vi "waveAquis.vi"(4 "Timeout (10000 ms)":u32=10000, 5 "Sub Channel(0: None)":u16(ring) items=["None", "SCH1", "SCH2", "SCH3", "SCH4", "SCH5", "SCH6", "SCH7", "SCH8", "SCH9", "SCH10", "SCH11", "SCH12", "SCH13", "SCH14", "SCH15", "SCH16", "SCH17", "SCH18", "SCH19", "SCH20", "SCH21", "SCH22", "SCH23", "SCH24", "SCH25", "SCH26", "SCH27", "SCH28", "SCH29", "SCH30", "SCH31", "SCH32", "SCH33", "SCH34", "SCH35", "SCH36", "SCH37", "SCH38", "SCH39", "SCH40", "SCH41", "SCH42", "SCH43", "SCH44", "SCH45", "SCH46", "SCH47", "SCH48", "SCH49", "SCH50", "SCH51", "SCH52", "SCH53", "SCH54", "SCH55", "SCH56", "SCH57", "SCH58", "SCH59", "SCH60", "SCH61", "SCH62", "SCH63", "SCH64"], 6 "End Point(1000)":i64=1000, 7 "Source (1: CH1)":i32(ring)=1 items=["", "CH1", "CH2", "CH3", "CH4", "CH5", "CH6", "CH7", "CH8", "CH9", "CH10", "CH11", "CH12", "CH13", "CH14", "CH15", "CH16", "MATH1", "MATH2", "MATH3", "MATH4", "MATH5", "MATH6", "MATH7", "MATH8", "EVENT"], 8 "error in (no error)":errorcluster, 9 "Start Point(0)":i64, 10 "Record Number (0)":i32, 11 "VISA resource name":refnum<visa-resource-name>) -> (0 "error out":errorcluster, 2 "Waveform Data":waveform(dbl)(graph), 3 "VISA resource name out":refnum<visa-resource-name>)   [LabVIEW 2019]
panel:
  out "read buffer":string
  out "output 2":dbl
  out "output 1":dbl
  out "1/x":dbl
  out "error out 9":errorcluster
  out "error out 8":errorcluster
  out "error out 7":errorcluster
  out "error out 6":errorcluster
  out "error out 5":errorcluster
  out "error out 4":errorcluster
  out "error out 3":errorcluster
  out "result":bool
  out "error out 2":errorcluster
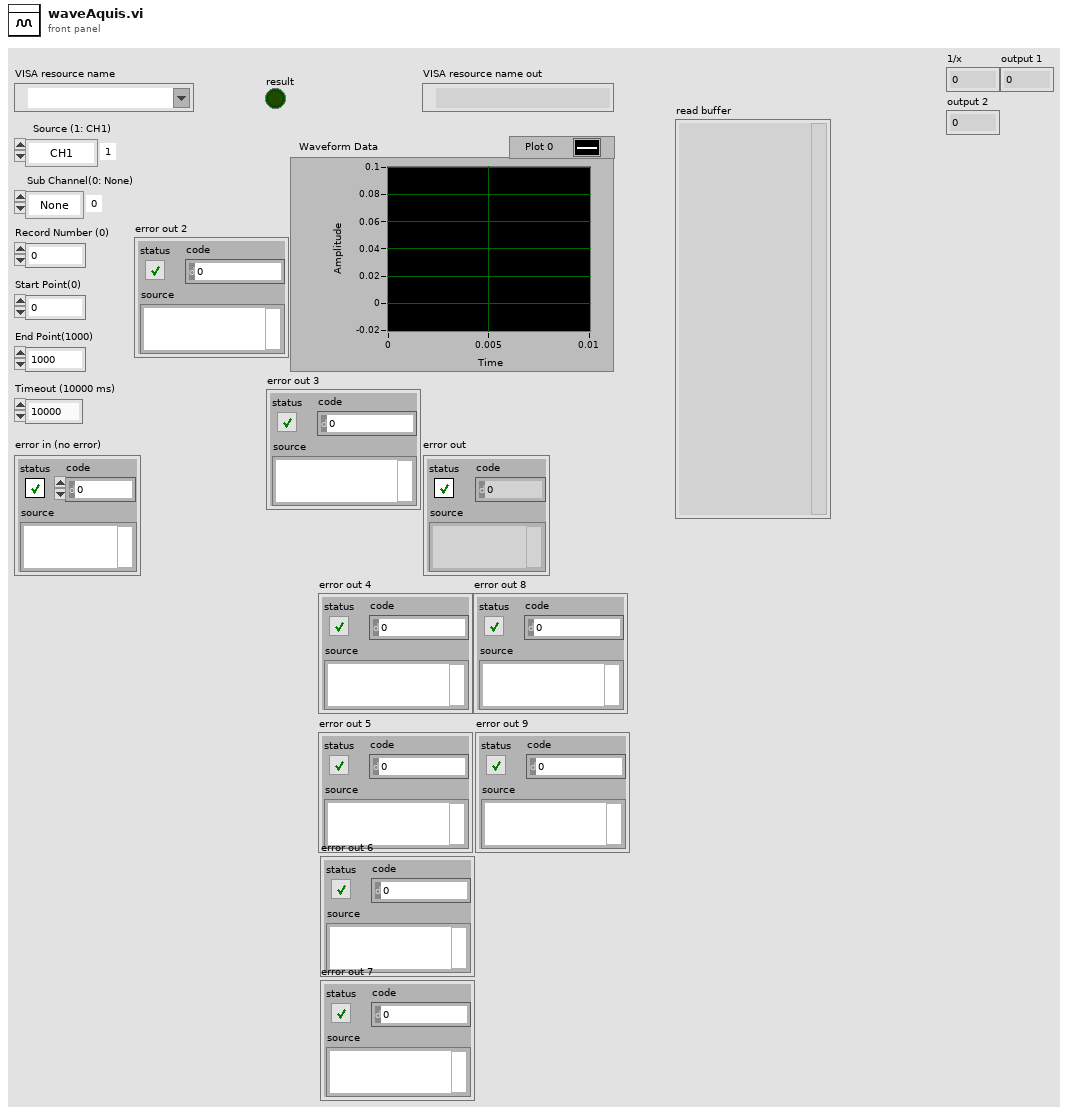
[diagram p1: front panel]
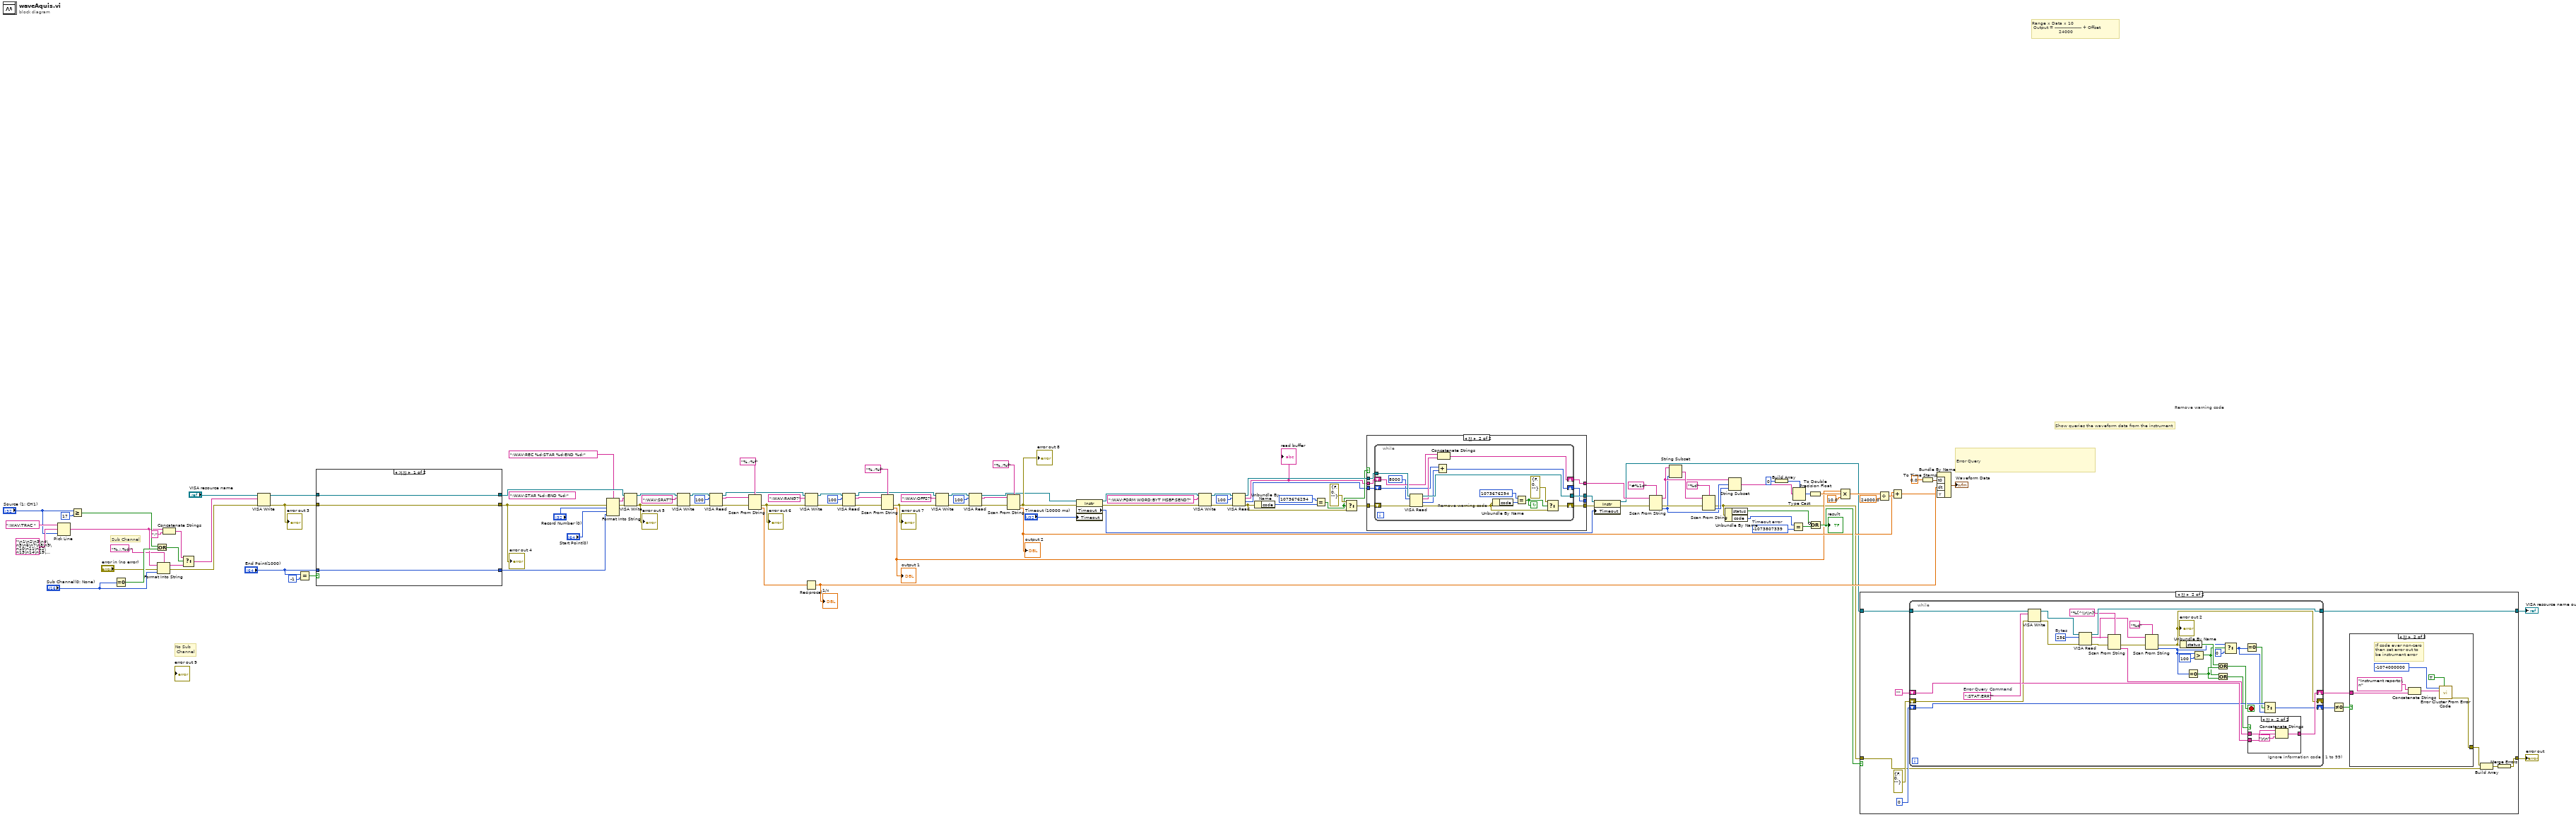
[diagram p0: block diagram]
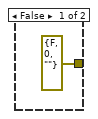
[diagram p4: hidden frame]
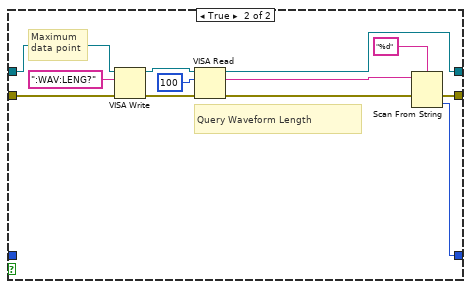
[diagram p6: hidden frame]
diagram:
  w61 = -1073807339  # Timeout error
  (unwired) ":WAV:STAR %d;:END %d;"
  # "Remove warning code"
  # "Show queries the waveform data from the instrument"
  # "Range x Data x 10\n Output = ------------------- + Offset \n                   24000"
  # "Error Query"
  # "Sub Channel"
  # "No Sub\n Channel"
  n1 = Pick Line ("ライン選択")(string ("")=":WAV:TRAC ", multi-line string="\n1\n2\n3\n4\n5\n6\n7\n8\n9\n10\n11\n12\n13\n14\n15\n16\nMATH1\nMATH2\nMATH3\nMATH4\nMATH5\nMATH6\nMATH7\nMATH8\nEVEN", line index="Source (1: CH1)") -> (output string=w95:string)
  n2 = Greater Or Equal? ("Èã?")(x="Source (1: CH1)", y=u16 17) -> (x >= y?=w109:bool)
  n3 = Equal To 0? ("0に等しい?")(x="Sub Channel(0: None)") -> (x = 0?=w110:bool)
  n4 = Or(x=w109, y=w110) -> (x .or. y?=w96:bool)
  n5 = Format Into String ("文字列にフォーマット")(format string="%.;,%d;", initial string=w95, error in="error in (no error)", "Sub Channel(0: None)") -> (resulting string=w93:string, error out=w101:errorcluster)
  n6 = Concatenate Strings ("•¶Žš—ñ˜AŒ‹")(w95, ";") -> (w97:string)
  n7 = Select(t=w97, s=w96, f=w93) -> (s? t:f=w92:string)
  n8 = VISA Write ("VISA書き込み")(VISA resource name="VISA resource name", write buffer=w92, error in (no error)=w101) -> (VISA resource name out=w100:refnum<visa-resource-name>, error out=w99:errorcluster)  [unwired: 1 out]
  "error out 3" <- w99
  n9 = Equal?(x="End Point(1000)", y=-1) -> (x = y?=w105:bool)
  n10 = case shown="거짓" w105 {
    tunnel: w100 -> [w115 w121]
    tunnel: [w115 w119] -> w104
    tunnel: [w116 w117] -> w103
    tunnel: "End Point(1000)" -> [w116 _]
    tunnel: w99 -> [w114 w120]
    tunnel: [w114 w118] -> w55
    frame False {
    }
    frame True {
      # "Query Waveform Length"
      # "Maximum\ndata point"
      n11 = VISA Write ("VISA書き込み")(VISA resource name=w121, write buffer=":WAV:LENG?", error in (no error)=w120) -> (VISA resource name out=w127:refnum<visa-resource-name>, error out=w128:errorcluster)  [unwired: 1 out]
      n12 = VISA Read ("VISA読み取り")(VISA resource name=w127, byte count=u32 100, error in (no error)=w128) -> (VISA resource name out=w119:refnum<visa-resource-name>, read buffer=w123:string, error out=w122:errorcluster)  [unwired: 1 out]
      n13 = Scan From String ("文字列からスキャン")(format string="%d", input string=w123, error in=w122) -> (error out=w118:errorcluster, output 1=w117:i32)  [unwired: 2 in, 2 out]
    }
  }
  "error out 4" <- w55
  n14 = Format Into String ("文字列にフォーマット")(format string=":WAV:REC %d;STAR %d;END %d;", error in=w55, "Record Number (0)", "Start Point(0)", w103) -> (resulting string=w4:string, error out=w5:errorcluster)  [unwired: 1 in]
  n15 = VISA Write ("VISA書き込み")(VISA resource name=w104, write buffer=w4, error in (no error)=w5) -> (VISA resource name out=w63:refnum<visa-resource-name>, error out=w54:errorcluster)  [unwired: 1 out]
  "error out 5" <- w54
  n16 = VISA Write ("VISA書き込み")(VISA resource name=w63, write buffer=":WAV:SRAT?", error in (no error)=w54) -> (VISA resource name out=w84:refnum<visa-resource-name>, error out=w86:errorcluster)  [unwired: 1 out]
  n17 = VISA Read ("VISA読み取り")(VISA resource name=w84, byte count=u32 100, error in (no error)=w86) -> (VISA resource name out=w62:refnum<visa-resource-name>, read buffer=w80:string, error out=w79:errorcluster)  [unwired: 1 out]
  n18 = Scan From String ("文字列からスキャン")(format string="%.;%f", input string=w80, error in=w79) -> (error out=w53:errorcluster, output 1=w81:dbl)  [unwired: 2 in, 2 out]
  "error out 6" <- w53
  n19 = VISA Write ("VISA書き込み")(VISA resource name=w62, write buffer=":WAV:RANG?", error in (no error)=w53) -> (VISA resource name out=w76:refnum<visa-resource-name>, error out=w77:errorcluster)  [unwired: 1 out]
  n20 = Reciprocal ("t")(x=w81) -> (1/x=w78:dbl)
  "1/x" <- w78
  n21 = VISA Read ("VISA読み取り")(VISA resource name=w76, byte count=u32 100, error in (no error)=w77) -> (VISA resource name out=w56:refnum<visa-resource-name>, read buffer=w72:string, error out=w71:errorcluster)  [unwired: 1 out]
  n22 = Scan From String(format string="%.;%f", input string=w72, error in=w71) -> (error out=w52:errorcluster, output 1=w34:dbl)  [unwired: 2 in, 2 out]
  "error out 7" <- w52
  "output 1" <- w34
  n23 = VISA Write ("VISA書き込み")(VISA resource name=w56, write buffer=":WAV:OFFS?", error in (no error)=w52) -> (VISA resource name out=w68:refnum<visa-resource-name>, error out=w70:errorcluster)  [unwired: 1 out]
  n24 = VISA Read ("VISA読み取り")(VISA resource name=w68, byte count=u32 100, error in (no error)=w70) -> (VISA resource name out=w17:refnum<visa-resource-name>, read buffer=w65:string, error out=w64:errorcluster)  [unwired: 1 out]
  n25 = Scan From String ("文字列からスキャン")(format string="%.;%f", input string=w65, error in=w64) -> (error out=w32:errorcluster, output 1=w35:dbl)  [unwired: 2 in, 2 out]
  "error out 8" <- w32
  "output 2" <- w35
  n26 = property on="プロパティノード" class="Instr"(reference=w17, error in=w32, "Timeout"="Timeout (10000 ms)") -> (reference out=w16:refnum<visa-resource-name>, error out=w11:errorcluster, "Timeout"=w33:u32)
  n27 = VISA Write(VISA resource name=w16, write buffer=":WAV:FORM WORD;BYT MSBF;SEND?", error in (no error)=w11) -> (VISA resource name out=w31:refnum<visa-resource-name>, error out=w30:errorcluster)  [unwired: 1 out]
  n28 = VISA Read(VISA resource name=w31, byte count=u32 100, error in (no error)=w30) -> (VISA resource name out=w29:refnum<visa-resource-name>, read buffer=w20:string, return count=w21:u32, error out=w24:errorcluster)
  "read buffer" <- w20
  n29 = Unbundle By Name(w24) -> ("code"=w28:i32)
  n30 = Equal?(x=1073676294, y=w28) -> (x = y?=w23:bool)
  n31 = Select(t=errorcluster {"status"=FALSE, "code"=0, "source"=""}, s=w23, f=w24) -> (s? t:f=w25:errorcluster)
  n32 = case shown="참" w23 {
    tunnel: w29 -> [w132 w140]
    tunnel: w25 -> [w131 w137]
    tunnel: [w132 w139] -> w19
    tunnel: [w131 w138] -> w18
    tunnel: w21 -> [w129 w136]
    tunnel: [w130 w135] -> w14
    tunnel: w20 -> [w130 w134]
    tunnel: [w129 w133] -> _
    frame False {
    }
    frame True {
      n33 = while {
        shift-left: w137 -> [w151]
        shift-right: [w142] -> w138
        shift-left: w134 -> [w153]
        shift-right: [w154] -> w135
        shift-left: w136 -> [w150]
        shift-right: [w148] -> w133
        tunnel: [w155] -> w139
        tunnel: w140 -> [w156]
        stop <- w141 continue-if-true
        # "Remove warning code"
        n34 = VISA Read(VISA resource name=w156, byte count=u32 8000, error in (no error)=w151) -> (VISA resource name out=w155:refnum<visa-resource-name>, read buffer=w152:string, return count=w149:u32, error out=w143:errorcluster)
        n35 = Add(x=w150, y=w149) -> (x+y=w148:u32)
        n36 = Concatenate Strings(w153, w152) -> (w154:string)
        n37 = Unbundle By Name(w143) -> ("code"=w146:i32)
        n38 = Equal?(x=1073676294, y=w146) -> (x = y?=w141:bool)
        n39 = Select(t=errorcluster {"status"=FALSE, "code"=0, "source"=""}, s=w141, f=w143) -> (s? t:f=w142:errorcluster)
      }
    }
  }
  n40 = property on="プロパティノード" class="Instr"(reference=w19, error in=w18, "Timeout"=w33) -> (reference out=w10:refnum<visa-resource-name>, error out=w9:errorcluster)
  n41 = Scan From String ("文字列からスキャン")(format string="#%1d", input string=w14, error in=w9) -> (remaining string=w40:string, error out=w45:errorcluster, output 1=w39:i32)  [unwired: 2 in, 1 out]
  n42 = String Subset ("•”•ª•¶Žš—ñ")(string=w40, length (rest)=w39) -> (substring=w42:string)  [unwired: 1 in]
  n43 = Scan From String ("文字列からスキャン")(format string="%d", input string=w42, error in=w45) -> (error out=w6:errorcluster, output 1=w41:i32)  [unwired: 2 in, 2 out]
  n44 = Unbundle By Name ("名前でバンドル解除")(w6) -> ("status"=w8:bool, "code"=w7:i32)
  n45 = String Subset ("•”•ª•¶Žš—ñ")(string=w40, offset (0)=w39, length (rest)=w41) -> (substring=w50:string)
  n46 = Build Array ("”z—ñ˜AŒ‹’Ç‰Á")(i16 0) -> (w48:i16[])
  n47 = Equal? ("等しい?")(x=w7, y=w61) -> (x = y?=w60:bool)
  n48 = Type Cast ("タイプキャスト")(type=w48, x=w50) -> (*(type *) &x=w51:i16[])
  n49 = To Double Precision Float ("倍精度浮動小数に変換")(number=w51) -> (double precision float=w38:dbl[])
  n50 = Compound Arithmetic op=OR ("¡Z")(invert w8, w60) -> (w59:bool)
  "result" <- w59
  n51 = Compound Arithmetic op=MULTIPLY(w34, w38, 10.0) -> (w36:dbl[])
  n52 = case "ケースストラクチャ" shown="참" w59 {
    tunnel: [w158 w170] -> w57
    tunnel: [w157 w168] -> w58
    tunnel: w10 -> [w158 w160]
    tunnel: w6 -> [w157 w159]
    frame False {
    }
    frame True {
      n53 = while "Whileループ" {
        tunnel: [w205] -> w170
        shift-right: [w196] -> w162
        shift-left: "" ("ó¶ñè") -> [w197]
        shift-right: [w194] -> w163
        shift-left: 0 -> [w195]
        shift-right: [w179] -> _
        shift-left: errorcluster {"status"=FALSE, "code"=0, "source"=""} ("error in (no error)") -> [w193]
        tunnel: w160 -> [w178]
        stop <- w200 stop-if-true
        w203 = u32 256  # Bytes
        w202 = ":STAT:ERR?"  # Error Query Command
        # "Ignore information code ( 1 to 99)"
        n54 = VISA Write ("VISA書き込み")(VISA resource name=w178, write buffer=w202, error in (no error)=w193) -> (VISA resource name out=w204:refnum<visa-resource-name>, error out=w180:errorcluster)  [unwired: 1 out]
        n55 = VISA Read ("VISA読み取り")(VISA resource name=w204, byte count=w203, error in (no error)=w180) -> (VISA resource name out=w205:refnum<visa-resource-name>, read buffer=w198:string, error out=w185:errorcluster)  [unwired: 1 out]
        n56 = Scan From String ("文字列からスキャン")(format string="%[^\\r\\n]", input string=w198, error in=w185) -> (error out=w192:errorcluster, output 1=w182:string)  [unwired: 2 in, 2 out]
        n57 = Scan From String ("文字列からスキャン")(format string="%d", input string=w198, error in=w192) -> (error out=w179:errorcluster, output 1=w189:i32)  [unwired: 2 in, 2 out]
        "error out 2" <- w179
        n58 = Unbundle By Name ("名前でバンドル解除")(w179) -> ("status"=w191:bool)
        n59 = Equal To 0? ("0に等しい?")(x=w189) -> (x = 0?=w184:bool)
        n60 = Greater? ("大きい?")(x=w189, y=100 ("x")) -> (0:w183:bool)
        n61 = Or(x=w191, y=w184) -> (x .or. y?=w200:bool)
        n62 = Or(x=w183, y=w184) -> (x .or. y?=w181:bool)
        n63 = Select ("‘I‘ð")(t=w189, s=w183, f=0) -> (s? t:f=w186:i32)
        n64 = Equal To 0? ("0に等しい?")(x=w186) -> (x = 0?=w187:bool)
        n65 = case "ケースストラクチャ" shown="참" w181 {
          tunnel: w197 -> [w206 w210]
          tunnel: [w206 w208] -> w196
          tunnel: w182 -> [_ w207]
          frame False {
          }
          frame True {
            n66 = Concatenate Strings ("•¶Žš—ñ˜AŒ‹")(w210, w207, "\r\n" ("Aüsè")) -> (w208:string)
          }
        }
        n67 = Select ("‘I‘ð")(t=w195, s=w187, f=w186) -> (s? t:f=w194:i32)
      }
      n68 = Not Equal To 0? ("0に等しくない?")(x=w163) -> (x != 0?=w166:bool)
      n69 = case "ケースストラクチャ" shown="참" w166 {
        tunnel: w162 -> [_ w176]
        tunnel: [errorcluster {"status"=FALSE, "code"=0, "source"=""} ("error out") w172] -> w165
        frame False {
        }
        frame True {
          # "If code ever non-zero\nthen set error out to\nbe instrument error"
          n70 = Concatenate Strings ("•¶Žš—ñ˜AŒ‹")("Instrument reports:\n" ("Source"), w176) -> (w173:string)
          n71 = call <vilib>:"Error Cluster From Error Code.vi"("show call chain? (False)"=TRUE, "error message (\"\")"=w173, "error code (0)"=-1074000000 ("Code")) -> ("error out"=w172:errorcluster)  [unwired: 6 in]
        }
      }
      n72 = Build Array(w165, w159) -> (w161:errorcluster[])
      n73 = Merge Errors(w161) -> (w168:errorcluster)
    }
  }
  "error out" <- w58
  "VISA resource name out" <- w57
  n74 = Divide ("¤")(x=w36, y=24000.0) -> (x/y=w46:dbl[])
  n75 = Add ("˜a")(x=w35, y=w46) -> (x+y=w13:dbl[])
  n76 = To Time Stamp ("タイムスタンプに変換")(1:0.0 ("l")) -> (0:w113:timestamp)
  n77 = Bundle By Name ("g`ì¬")("t0"=w113, "dt"=w78, "Y"=w13) -> (→"Waveform Data":waveform(dbl))  [unwired: 1 in]
